vi "getVcselPulsePeriod.vi"(8 "error in":errorcluster, 9 "vcselPeriodType":T9(ring), 10 "Slave Address (7-bit)":u8, 11 "I2C Ref In":T1) -> (0 "error out":errorcluster, 2 "VcselPulsePeriod":u8, 3 "I2C Ref Out":T1)   [LabVIEW 2018]
uses:
  <vilib>/myRIO/Instrument Drivers/Onboard IO/I2C/typedefs/I2C Reference.ctl
  <vilib>/myRIO/Common/Instrument Driver Framework/Utilities/typedefs/myRIO Generic Hardware Reference.ctl
  <vilib>/myRIO/Common/Instrument Driver Framework/Utilities/typedefs/Hardware Version Enum.ctl
  <vilib>/myRIO/Common/Instrument Driver Framework/Utilities/typedefs/myRIO v1.0 Reference.ctl
  <vilib>/myRIO/Common/Instrument Driver Framework/Utilities/typedefs/Generic FPGA Reference.ctl
  <vilib>/myRIO/Common/Instrument Driver Framework/myRIO v1.0/I2C/typedefs/I2C Channels Enum.ctl
  <vilib>/myRIO/Instrument Drivers/Onboard IO/I2C/typedefs/I2C Configuration.ctl
  <vilib>/myRIO/Instrument Drivers/Onboard IO/I2C/typedefs/I2C Transfer Rate.ctl
  <vilib>/Utility/error.llb/Error Cluster From Error Code.vi
  <vilib>/myRIO/Common/Instrument Driver Framework/myRIO v1.0/I2C/vis/myRIO v1.0 Write I2C.vi
  <vilib>/myRIO/Common/Instrument Driver Framework/myRIO v1.0/I2C/vis/myRIO v1.0 Read I2C.vi
  <vilib>/myRIO/Instrument Drivers/Onboard IO/I2C/I2C.lvlib
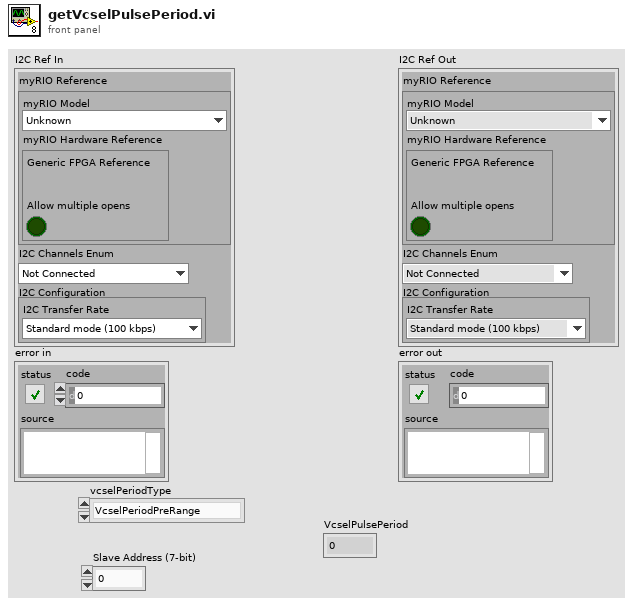
[diagram p1: front panel]
types:
  T1 = typedef "I2C.lvlib/I2C Reference.ctl" = cluster{"myRIO Reference":T2, "I2C Channels Enum":T6, "I2C Configuration":T7}
  T2 = typedef "myRIO Generic Hardware Reference.ctl" = cluster{"myRIO Model":T3, "myRIO Hardware Reference":T4}
  T3 = typedef "Hardware Version Enum.ctl" = enum16{"Unknown", "myRIO-1900", "myRIO-1950", "roboRIO", "NI ELVIS RIO CM", "ELVIS III"}
  T4 = typedef "myRIO v1.0 Reference.ctl" = cluster{"Generic FPGA Reference":T5, "Allow multiple opens":bool}
  T5 = typedef "Generic FPGA Reference.ctl" = refnum<k20>
  T6 = typedef "I2C Channels Enum.ctl" = enum16{"Not Connected", "A/I2C", "B/I2C", "I2C/I2C"}
  T7 = typedef "I2C.lvlib/I2C Configuration.ctl" = cluster{"I2C Transfer Rate":T8}
  T8 = typedef "I2C.lvlib/I2C Transfer Rate.ctl" = enum16{"Standard mode (100 kbps)", "Fast mode (400 kbps)"}
  T9 = enum8{"VcselPeriodPreRange", "VcselPeriodFinalRange"}
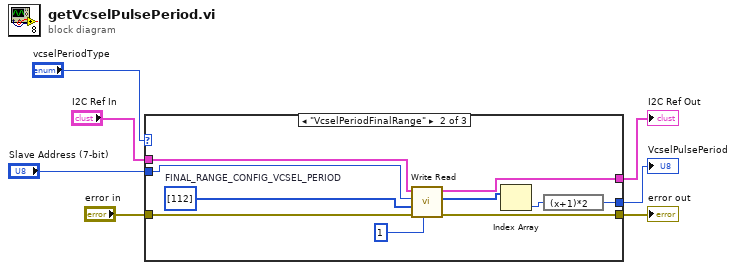
[diagram p0: block diagram]
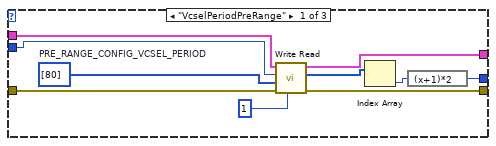
[diagram p2: hidden frame]
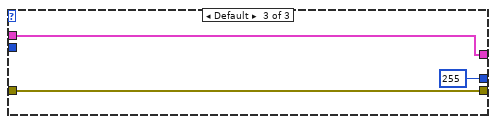
[diagram p3: hidden frame]
diagram:
  n1 = case shown="\"VcselPeriodFinalRange\"" "vcselPeriodType" {
    tunnel: [w8 w18 u8 255] -> w1
    tunnel: "Slave Address (7-bit)" -> [w17 w23 _]
    tunnel: "I2C Ref In" -> [w16 w24 w29]
    tunnel: [w15 w25 w29] -> w4
    tunnel: [w14 w26 w28] -> w3
    tunnel: "error in" -> [w13 w27 w28]
    frame "VcselPeriodPreRange" {
      w10 = u8[] [80]  # PRE_RANGE_CONFIG_VCSEL_PERIOD
      n2 = call <vilib>:"Write Read.vi"("Byte Count"=u32 1, "error in (no error)"=w13, "Bytes to Write"=w10, "Slave Address (7-bit)"=w17, "I2C Ref In"=w16) -> ("error out"=w14:errorcluster, "Bytes Read"=w12:u8[], "I2C Ref Out"=w15:T1)  [unwired: 3 in]
      n3 = Index Array(array=w12) -> (element=w9:u8)  [unwired: 1 in]
      n4 = expression code="(x+1)*2"(w9) -> (w8:u8)
    }
    frame "VcselPeriodFinalRange" {
      w21 = u8[] [112]  # FINAL_RANGE_CONFIG_VCSEL_PERIOD
      n5 = call <vilib>:"Write Read.vi"("Byte Count"=u32 1, "error in (no error)"=w27, "Bytes to Write"=w21, "Slave Address (7-bit)"=w23, "I2C Ref In"=w24) -> ("error out"=w26:errorcluster, "Bytes Read"=w20:u8[], "I2C Ref Out"=w25:T1)  [unwired: 3 in]
      n6 = Index Array(array=w20) -> (element=w19:u8)  [unwired: 1 in]
      n7 = expression code="(x+1)*2"(w19) -> (w18:u8)
    }
    frame Default {
    }
  }
  "error out" <- w3
  "I2C Ref Out" <- w4
  "VcselPulsePeriod" <- w1
